vi "Close.vi"(8 "Error In":errorcluster, 11 "Keithley 2602 In":refnum<visa-resource-name>) -> (0 "Error Out":errorcluster)   [LabVIEW 2013, in "Keithley-2602.lvlib"]
uses:
  Keithley-2602.lvlib
  Controls/DisplayScreen.ctl
  Controls/SMU.ctl
  Controls/DisplayFunction.ctl
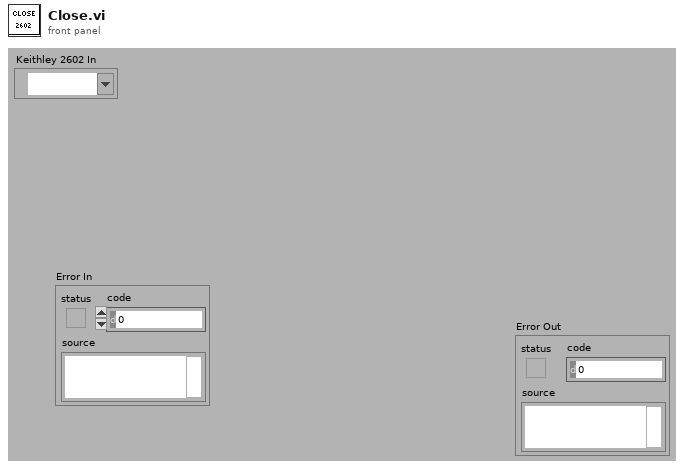
[diagram p1: front panel]
types:
  T1 = typedef "Keithley-2602.lvlib/SMU.ctl" = enum16{"A", "B"}
  T2 = typedef "Keithley-2602.lvlib/DisplayFunction.ctl" = enum16{"Current", "Voltage", "Resistance", "Power"}
  T3 = typedef "Keithley-2602.lvlib/DisplayScreen.ctl" = enum16{"SMU A", "SMU B", "Both", "User"}
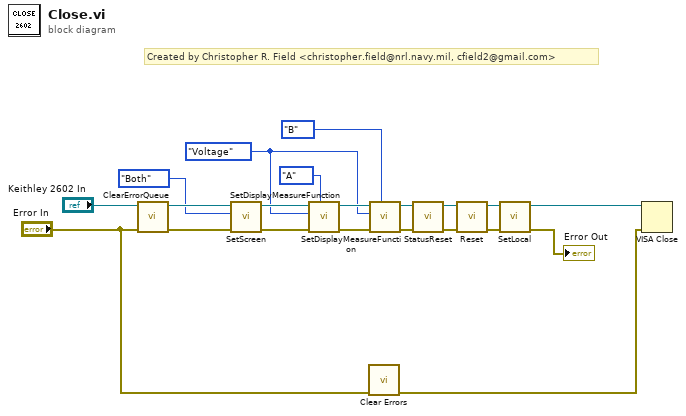
[diagram p0: block diagram]
diagram:
  w5 = DisplayFunction."Voltage" ("Display Function")
  # "Created by Christopher R. Field <christopher.field@nrl.navy.mil, cfield2@gmail.com>"
  n1 = call "ClearErrorQueue.vi"("Error In"="Error In", "Keithley 2602 In"="Keithley 2602 In") -> ("Error Out"=w13:errorcluster, "Keithley 2602 Out"=w14:refnum<visa-resource-name>)  [unwired: 8 in]
  n2 = call "SetScreen.vi"("Error In"=w13, "Display Screen"=DisplayScreen."Both", "Keithley 2602 In"=w14) -> ("Error Out"=w19:errorcluster, "Keithley 2602 Out"=w20:refnum<visa-resource-name>)  [unwired: 7 in]
  n3 = call "SetDisplayMeasureFunction.vi"("SMU"=SMU."A", "Error In"=w19, "Display Function"=w5, "Keithley 2602 In"=w20) -> ("Error Out"=w17:errorcluster, "Keithley 2602 Out"=w18:refnum<visa-resource-name>)  [unwired: 6 in]
  n4 = call <vilib>:"Clear Errors.vi"("error in (no error)"="Error In") -> ("error out"=w1:errorcluster)  [unwired: 6 in]
  n5 = call "SetDisplayMeasureFunction.vi"("SMU"=SMU."B", "Error In"=w17, "Display Function"=w5, "Keithley 2602 In"=w18) -> ("Error Out"=w9:errorcluster, "Keithley 2602 Out"=w11:refnum<visa-resource-name>)  [unwired: 6 in]
  n6 = call "StatusReset.vi"("Error In"=w9, "Keithley 2602 In"=w11) -> ("Error Out"=w8:errorcluster, "Keithley 2602 Out"=w10:refnum<visa-resource-name>)  [unwired: 8 in]
  n7 = call "Reset.vi"("Error In"=w8, "Keithley 2602 In"=w10) -> ("Error Out"=w15:errorcluster, "Keithley 2602 Out"=w16:refnum<visa-resource-name>)  [unwired: 8 in]
  n8 = call "SetLocal.vi"("Error In"=w15, "Keithley 2602 In"=w16) -> ("Error Out"=→"Error Out":errorcluster, "Keithley 2602 Out"=w21:refnum<visa-resource-name>)  [unwired: 8 in]
  n9 = VISA Close(VISA resource name=w21, error in (no error)=w1) -> ()  [unwired: 1 out]
